vi "Angle.vi"(8 "Angle":dbl[][](array[numeric])) -> (0 "Shoulder-Elbow angle data":dbl[][](array[numeric]), 1 "Pos, Neg increments":dbl[][](array[numeric]), 2 "Elbow CircStat":dbl[](array[numeric]), 3 "Shoulder CircStat Counterclockwise":dbl[](array[numeric]), 4 "Angle mean subtracted (output)":dbl[][](array[numeric]), 5 "Angle RMS":dbl[][](array[numeric]), 6 "Angle for Synergy analysis":dbl[][](array[numeric]))   [LabVIEW 2020]
uses:
  <vilib>/Analysis/baseanly.llb/Mean (DBL).vi
  <vilib>/Analysis/5stat.llb/RMS (DBL).vi
  <vilib>/Analysis/NI_AALBase.lvlib
  <vilib>/Analysis/NI_AALPro.lvlib
panel:
  out "Shoulder-Elbow angle data":dbl[](array[numeric])
  out "Elbow joint angle CircStats 2":dbl[](graph)
  out "size(s) 2":i32
  out "Elbow Flexion":dbl
  out "Negative increments":dbl[](array[numeric])
  out "Elbow Extension":dbl
  out "Positive increments":dbl[](array[numeric])
  out "size(s)":i32
  out "Shoulder Flexion":dbl
  out "Negative increments":dbl[](array[numeric])
  out "Shoulder Extension":dbl
  out "Positive increments":dbl[](array[numeric])
  out "Elbow joint angle CircStats":dbl[](graph)
  out "Shoulder joint angle CircStats CounterClockwise":dbl[](graph)
  out "Elbow Angle Circular correction Clockwise":dbl[](array[numeric])
  out "floor(x): largest int <= x 2":dbl
  out "Shoulder angle Circular correction CounterClockwise":dbl[](array[numeric])
  out "Shoulder angle Circular correction Clockwise":dbl[](array[numeric])
  out "floor(x): largest int <= x":dbl
  out "Elbow Angle (output)":dbl[](array[numeric])
  out "Elbow joint angle":dbl[](graph)
  out "Shoulder Angle (output)":dbl[](array[numeric])
  out "Shoulder joint angle":dbl[](graph)
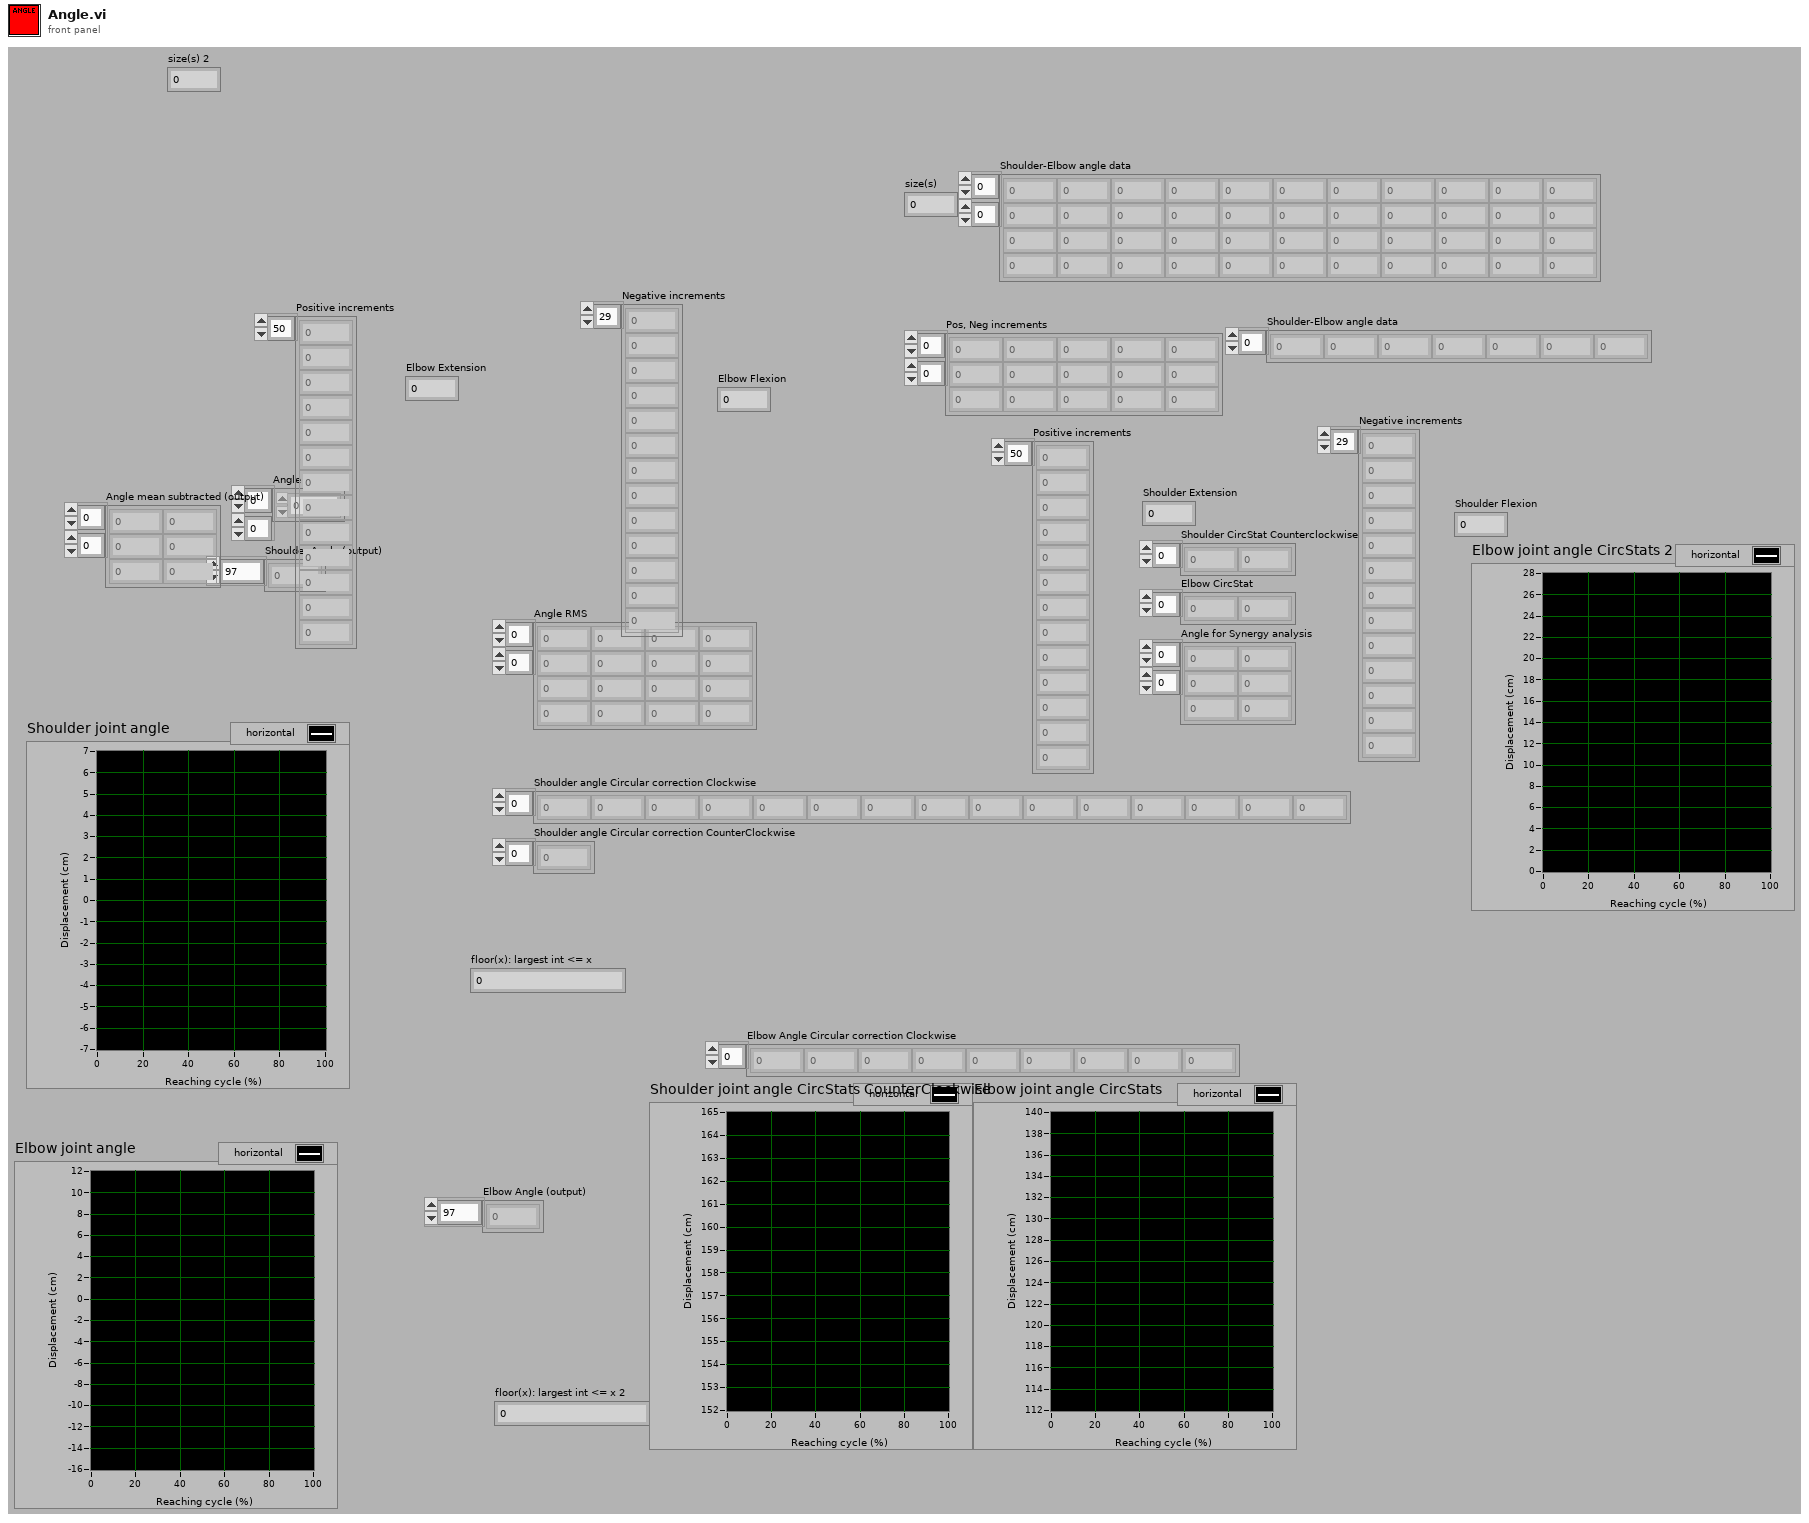
[diagram p1: front panel]
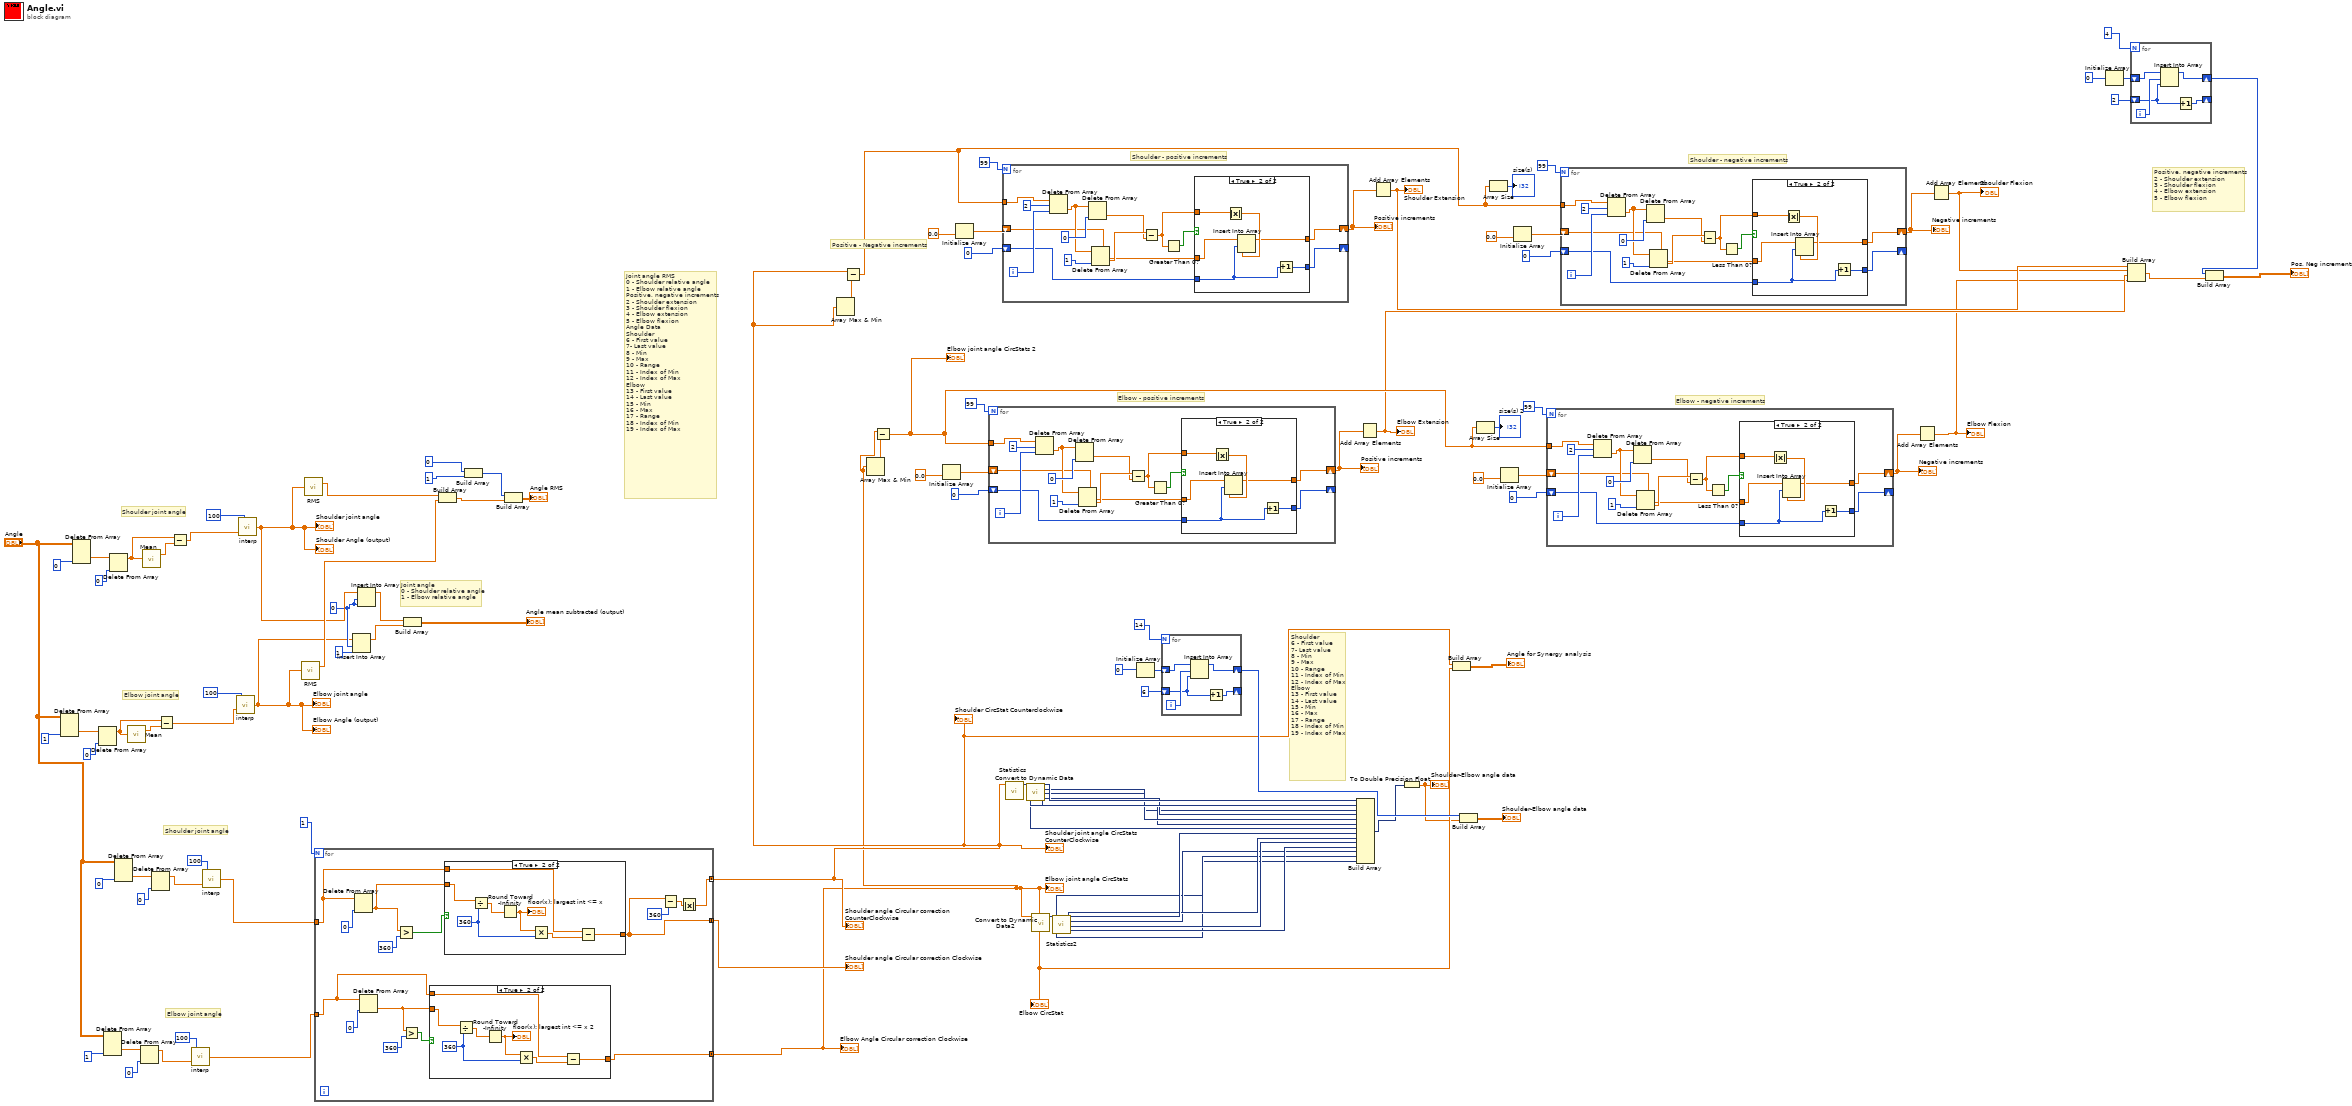
[diagram p0: block diagram]
diagram:
  w21 = 0
  # "Joint angle RMS\n0 - Shoulder relative angle\n1 - Elbow relative angle\nPositive, negative increments\n2 - Shoulder extension\n3 - Shoulder flexion\n4 - Elbow extension\n5 - Elbow flexion\nAngle Data\nShoulder\n6 - First value\n7- Last value\n8 - Min\n9 - Max\n10 - Range\n11 - Index of Min\n12 - Index of Max\nElbow\n13 - First value\n14 - Last value\n15 - Min\n16 - Max\n17 - Range\n18 - Index of Min\n19 - Index of Max"
  # "Positive, negative increments\n2 - Shoulder extension\n3 - Shoulder flexion\n4 - Elbow extension\n5 - Elbow flexion"
  # "Elbow - negative increments"
  # "Elbow - positive increments"
  # "Shoulder - negative increments"
  # "Shoulder - positive increments"
  # "Positive - Negative increments"
  # "Shoulder\n6 - First value\n7- Last value\n8 - Min\n9 - Max\n10 - Range\n11 - Index of Min\n12 - Index of Max\nElbow\n13 - First value\n14 - Last value\n15 - Min\n16 - Max\n17 - Range\n18 - Index of Min\n19 - Index of Max"
  # "Elbow joint angle"
  # "Shoulder joint angle"
  # "Joint angle\n0 - Shoulder relative angle\n1 - Elbow relative angle"
  # "Elbow joint angle"
  # "Shoulder joint angle"
  n1 = Delete From Array(array="Angle", index (col)=1) -> (deleted portion=w96:dbl[])  [unwired: 2 in, 1 out]
  n2 = Delete From Array(array="Angle", index (col)=0) -> (deleted portion=w103:dbl[])  [unwired: 2 in, 1 out]
  n3 = Delete From Array(array=w96, index=0) -> (array with subset deleted=w94:dbl[])  [unwired: 1 in, 1 out]
  n4 = Delete From Array(array="Angle", index (col)=1) -> (deleted portion=w79:dbl[])  [unwired: 2 in, 1 out]
  n5 = Delete From Array(array=w103, index=0) -> (array with subset deleted=w101:dbl[])  [unwired: 1 in, 1 out]
  n6 = Delete From Array(array="Angle", index (col)=0) -> (deleted portion=w83:dbl[])  [unwired: 2 in, 1 out]
  n7 = call-poly <vilib>:"Mean.vi"("X"=w94) -> ("mean"=w99:dbl)  [unwired: 1 out]
  n8 = Delete From Array(array=w79, index=0) -> (array with subset deleted=w76:dbl[])  [unwired: 1 in, 1 out]
  n9 = call-poly <vilib>:"Mean.vi"("X"=w101) -> ("mean"=w106:dbl)  [unwired: 1 out]
  n10 = Delete From Array(array=w83, index=0) -> (array with subset deleted=w75:dbl[])  [unwired: 1 in, 1 out]
  n11 = Subtract(x=w94, y=w99) -> (x-y=w97:dbl[])
  n12 = Subtract(x=w101, y=w106) -> (x-y=w104:dbl[])
  n13 = call "interp.vi"("first subarray"=w76, "nFRAMES"=100) -> ("emgInterp"=w71:dbl[])
  n14 = call "interp.vi"("first subarray"=w75, "nFRAMES"=100) -> ("emgInterp"=w72:dbl[])
  n15 = call "interp.vi"("first subarray"=w97, "nFRAMES"=100) -> ("emgInterp"=w17:dbl[])
  "Elbow joint angle" <- w17
  "Elbow Angle (output)" <- w17
  n16 = call "interp.vi"("first subarray"=w104, "nFRAMES"=100) -> ("emgInterp"=w22:dbl[])
  "Shoulder joint angle" <- w22
  "Shoulder Angle (output)" <- w22
  n17 = call-poly <vilib>:"RMS.vi"("X"=w17) -> ("rms value"=w91:dbl)  [unwired: 1 out]
  n18 = call-poly <vilib>:"RMS.vi"("X"=w22) -> ("rms value"=w92:dbl)  [unwired: 1 out]
  n19 = for {
    N: 1 -> [_]
    tunnel: w72 -> [w118]
    tunnel: [w117] -> w74 mode=concatenating
    tunnel: [w114] -> w5 mode=concatenating
    tunnel: w71 -> [w111]
    tunnel: [w109] -> w4 mode=concatenating
    n20 = Delete From Array(array=w118, index=0) -> (deleted portion=w119:dbl)  [unwired: 1 in, 1 out]
    n21 = Delete From Array(array=w111, index=0) -> (deleted portion=w110:dbl)  [unwired: 1 in, 1 out]
    n22 = Greater?(x=w119, y=360) -> (0:w120:bool)
    n23 = Greater?(x=w110, y=360) -> (0:w108:bool)
    n24 = case shown="True" w108 {
      tunnel: w110 -> [_ w130]
      tunnel: w111 -> [w123 w126]
      tunnel: [w123 w124] -> w109
      frame False {
      }
      frame True {
        w127 = 360
        n25 = Divide(x=w130, y=w127) -> (x/y=w129:dbl)
        n26 = Round Toward -Infinity(1:w129) -> (0:w128:dbl)
        "floor(x): largest int <= x 2" <- w128
        n27 = Multiply(x=w128, y=w127) -> (x*y=w125:dbl)
        n28 = Subtract(x=w126, y=w125) -> (x-y=w124:dbl[])
      }
    }
    n29 = case shown="True" w120 {
      tunnel: w119 -> [_ w138]
      tunnel: w118 -> [w131 w134]
      tunnel: [w131 w132] -> w117
      frame False {
      }
      frame True {
        w135 = 360
        n30 = Divide(x=w138, y=w135) -> (x/y=w137:dbl)
        n31 = Round Toward -Infinity(1:w137) -> (0:w136:dbl)
        "floor(x): largest int <= x" <- w136
        n32 = Multiply(x=w136, y=w135) -> (x*y=w133:dbl)
        n33 = Subtract(x=w134, y=w133) -> (x-y=w132:dbl[])
      }
    }
    n34 = Subtract(x=w117, y=360) -> (x-y=w115:dbl[])
    n35 = Absolute Value(x=w115) -> (abs(x)=w114:dbl[])
  }
  "Shoulder angle Circular correction Clockwise" <- w74
  "Shoulder angle Circular correction CounterClockwise" <- w5
  "Elbow Angle Circular correction Clockwise" <- w4
  "Shoulder joint angle CircStats CounterClockwise" <- w5
  "Elbow joint angle CircStats" <- w4
  "Shoulder CircStat Counterclockwise" <- w5
  "Elbow CircStat" <- w4
  n36 = Insert Into Array(array=w17, index=w21, new element=1) -> (w18:dbl[])
  n37 = Insert Into Array(array=w22, index=w21, new element=w21) -> (w19:dbl[])
  n38 = Build Array(w19, w18) -> (→"Angle mean subtracted (output)":dbl[][])
  n39 = Build Array(w92, w91) -> (w87:dbl[])
  n40 = Build Array(0, 1) -> (w88:i32[])
  n41 = Build Array(w88, w87) -> (→"Angle RMS":dbl[][])
  n42 = Array Max & Min(array=w5) -> (min value=w54:dbl)  [unwired: 3 out]
  n43 = Subtract(x=w5, y=w54) -> (x-y=w43:dbl[])
  n44 = Array Max & Min(array=w4) -> (min value=w30:dbl)  [unwired: 3 out]
  n45 = Subtract(x=w4, y=w30) -> (x-y=w29:dbl[])
  "Elbow joint angle CircStats 2" <- w29
  n46 = Initialize Array(0.0) -> (w40:dbl[])  [unwired: 1 in]
  n47 = Initialize Array(0.0) -> (w52:dbl[])  [unwired: 1 in]
  n48 = for {
    N: 99 -> [_]
    shift-right: [w139] -> _
    shift-left: 0 -> [w141]
    shift-right: [w140] -> w37
    shift-left: w40 -> [w142]
    tunnel: w29 -> [w152]
    i -> [w151]
    n49 = Delete From Array(array=w152, length=2, index=w151) -> (deleted portion=w147:dbl[])  [unwired: 1 out]
    n50 = Delete From Array(array=w147, index=0) -> (deleted portion=w145:dbl)  [unwired: 1 in, 1 out]
    n51 = Delete From Array(array=w147, index=1) -> (deleted portion=w146:dbl)  [unwired: 1 in, 1 out]
    n52 = Subtract(x=w146, y=w145) -> (x-y=w143:dbl)
    n53 = Greater Than 0?(x=w143) -> (x > 0?=w144:bool)
    n54 = case shown="True" w144 {
      tunnel: w143 -> [_ w160]
      tunnel: w142 -> [w154 w159]
      tunnel: w141 -> [w153 w156]
      tunnel: [w154 w157] -> w140
      tunnel: [w153 w155] -> w139
      frame False {
      }
      frame True {
        n55 = Absolute Value(x=w160) -> (abs(x)=w158:dbl)
        n56 = Insert Into Array(array=w159, index=w156, new element=w158) -> (w157:dbl[])
        n57 = Increment(x=w156) -> (x+1=w155:i32)
      }
    }
  }
  "Positive increments" <- w37
  n58 = for {
    N: 99 -> [_]
    shift-right: [w161] -> _
    shift-left: 0 -> [w163]
    shift-right: [w162] -> w49
    shift-left: w52 -> [w164]
    tunnel: w43 -> [w174]
    i -> [w173]
    n59 = Delete From Array(array=w174, length=2, index=w173) -> (deleted portion=w169:dbl[])  [unwired: 1 out]
    n60 = Delete From Array(array=w169, index=0) -> (deleted portion=w167:dbl)  [unwired: 1 in, 1 out]
    n61 = Delete From Array(array=w169, index=1) -> (deleted portion=w168:dbl)  [unwired: 1 in, 1 out]
    n62 = Subtract(x=w168, y=w167) -> (x-y=w165:dbl)
    n63 = Greater Than 0?(x=w165) -> (x > 0?=w166:bool)
    n64 = case shown="True" w166 {
      tunnel: w165 -> [_ w182]
      tunnel: w164 -> [w176 w181]
      tunnel: w163 -> [w175 w178]
      tunnel: [w176 w179] -> w162
      tunnel: [w175 w177] -> w161
      frame False {
      }
      frame True {
        n65 = Absolute Value(x=w182) -> (abs(x)=w180:dbl)
        n66 = Insert Into Array(array=w181, index=w178, new element=w180) -> (w179:dbl[])
        n67 = Increment(x=w178) -> (x+1=w177:i32)
      }
    }
  }
  "Positive increments" <- w49
  n68 = call "Convert to Dynamic Data"("Array"=w5) -> ("Dynamic Data Type"=w70:dynamicdata)  [unwired: 3 in]
  n69 = call "Statistics"("Signals"=w70) -> ("Index of Max"=w63:dynamicdata, "Index of Min"=w64:dynamicdata, "Last Value"=w67:dynamicdata, "First Value"=w68:dynamicdata, "Range"=w65:dynamicdata, "Minimum"=w55:dynamicdata, "Maximum"=w66:dynamicdata)  [unwired: 19 in, 1 out]
  n70 = call "Convert to Dynamic Data2"("Array"=w4) -> ("Dynamic Data Type"=w69:dynamicdata)  [unwired: 3 in]
  n71 = call "Statistics2"("Signals"=w69) -> ("Index of Max"=w56:dynamicdata, "Index of Min"=w57:dynamicdata, "Last Value"=w61:dynamicdata, "First Value"=w62:dynamicdata, "Range"=w58:dynamicdata, "Minimum"=w60:dynamicdata, "Maximum"=w59:dynamicdata)  [unwired: 19 in, 1 out]
  n72 = Initialize Array(0) -> (w26:i32[])  [unwired: 1 in]
  n73 = for {
    N: 14 -> [_]
    shift-right: [w185] -> w24
    shift-left: w26 -> [w186]
    shift-right: [w183] -> _
    shift-left: 6 -> [w184]
    i -> [w187]
    n74 = Insert Into Array(array=w186, index=w187, new element=w184) -> (w185:i32[])
    n75 = Increment(x=w184) -> (x+1=w183:i32)
  }
  n76 = Build Array(w68, w67, w55, w66, w65, w64, w63, w62, w61, w60, w59, w58, w57, w56) -> (w2:dynamicdata[])
  n77 = Add Array Elements(numeric array=w37) -> (sum=w14:dbl)
  "Elbow Extension" <- w14
  n78 = Add Array Elements(numeric array=w49) -> (sum=w16:dbl)
  "Shoulder Extension" <- w16
  n79 = To Double Precision Float(number=w2) -> (double precision float=w1:dbl[])
  "Shoulder-Elbow angle data" <- w1
  n80 = Build Array(w5, w4) -> (→"Angle for Synergy analysis":dbl[][])
  n81 = Build Array(w24, w1) -> (→"Shoulder-Elbow angle data":dbl[][])
  n82 = Array Size(array=w29) -> (size(s)=→"size(s) 2":i32)
  n83 = Array Size(array=w43) -> (size(s)=→"size(s)":i32)
  n84 = Initialize Array(0.0) -> (w35:dbl[])  [unwired: 1 in]
  n85 = Initialize Array(0.0) -> (w47:dbl[])  [unwired: 1 in]
  n86 = for {
    N: 99 -> [_]
    shift-right: [w188] -> _
    shift-left: 0 -> [w190]
    shift-right: [w189] -> w32
    shift-left: w35 -> [w191]
    tunnel: w29 -> [w201]
    i -> [w200]
    n87 = Delete From Array(array=w201, length=2, index=w200) -> (deleted portion=w196:dbl[])  [unwired: 1 out]
    n88 = Delete From Array(array=w196, index=0) -> (deleted portion=w194:dbl)  [unwired: 1 in, 1 out]
    n89 = Delete From Array(array=w196, index=1) -> (deleted portion=w195:dbl)  [unwired: 1 in, 1 out]
    n90 = Subtract(x=w195, y=w194) -> (x-y=w192:dbl)
    n91 = Less Than 0?(x=w192) -> (x < 0?=w193:bool)
    n92 = case shown="True" w193 {
      tunnel: w192 -> [_ w209]
      tunnel: w191 -> [w203 w208]
      tunnel: w190 -> [w202 w205]
      tunnel: [w203 w206] -> w189
      tunnel: [w202 w204] -> w188
      frame False {
      }
      frame True {
        n93 = Absolute Value(x=w209) -> (abs(x)=w207:dbl)
        n94 = Insert Into Array(array=w208, index=w205, new element=w207) -> (w206:dbl[])
        n95 = Increment(x=w205) -> (x+1=w204:i32)
      }
    }
  }
  "Negative increments" <- w32
  n96 = for {
    N: 99 -> [_]
    shift-right: [w210] -> _
    shift-left: 0 -> [w212]
    shift-right: [w211] -> w44
    shift-left: w47 -> [w213]
    tunnel: w43 -> [w223]
    i -> [w222]
    n97 = Delete From Array(array=w223, length=2, index=w222) -> (deleted portion=w218:dbl[])  [unwired: 1 out]
    n98 = Delete From Array(array=w218, index=0) -> (deleted portion=w216:dbl)  [unwired: 1 in, 1 out]
    n99 = Delete From Array(array=w218, index=1) -> (deleted portion=w217:dbl)  [unwired: 1 in, 1 out]
    n100 = Subtract(x=w217, y=w216) -> (x-y=w214:dbl)
    n101 = Less Than 0?(x=w214) -> (x < 0?=w215:bool)
    n102 = case shown="True" w215 {
      tunnel: w214 -> [_ w231]
      tunnel: w213 -> [w225 w230]
      tunnel: w212 -> [w224 w227]
      tunnel: [w225 w228] -> w211
      tunnel: [w224 w226] -> w210
      frame False {
      }
      frame True {
        n103 = Absolute Value(x=w231) -> (abs(x)=w229:dbl)
        n104 = Insert Into Array(array=w230, index=w227, new element=w229) -> (w228:dbl[])
        n105 = Increment(x=w227) -> (x+1=w226:i32)
      }
    }
  }
  "Negative increments" <- w44
  n106 = Add Array Elements(numeric array=w32) -> (sum=w13:dbl)
  "Elbow Flexion" <- w13
  n107 = Add Array Elements(numeric array=w44) -> (sum=w15:dbl)
  "Shoulder Flexion" <- w15
  n108 = Initialize Array(0) -> (w10:i32[])  [unwired: 1 in]
  n109 = Build Array(w16, w15, w14, w13) -> (w7:dbl[])
  n110 = for {
    N: 4 -> [_]
    shift-right: [w234] -> w8
    shift-left: w10 -> [w235]
    shift-right: [w232] -> _
    shift-left: 2 -> [w233]
    i -> [w236]
    n111 = Insert Into Array(array=w235, index=w236, new element=w233) -> (w234:i32[])
    n112 = Increment(x=w233) -> (x+1=w232:i32)
  }
  n113 = Build Array(w8, w7) -> (→"Pos, Neg increments":dbl[][])
